vi "Print.vi"(5 "Orientation (0: Portrait)":i32(ring) items=["Portrait", "Landscape"], 7 "File Format (0: BMP)":i32(ring) items=["BMP", "Canon BubbleJet", "HP DeskJet", "Seiko DPU3445", "Seiko DPU411", "Seiko DPU412", "Epson C60", "Epson C80", "Epson Postscript", "Epson Dot Matrix", "Interleaf", "HP LaserJet II", "PCX", "RLE", "HP ThinkJet", "TIFF"], 8 "error in (no error)":errorcluster, 9 "Ink Saver (Off)":bool, 10 "Port (0: Centronics)":i32(ring) items=["Centronics", "Serial", "GPIB"], 11 "VISA resource name":refnum<visa-resource-name>) -> (0 "error out":errorcluster, 3 "VISA resource name out":refnum<visa-resource-name>)   [LabVIEW 2017, in "Tektronix TDS 200 1000 2000 Series.lvlib"]
doc: "Sets the format, orientation, and port for hardcopy printing."
uses:
  Tektronix TDS 200 1000 2000 Series.lvlib
panel:
  # "On"
  # "Off"
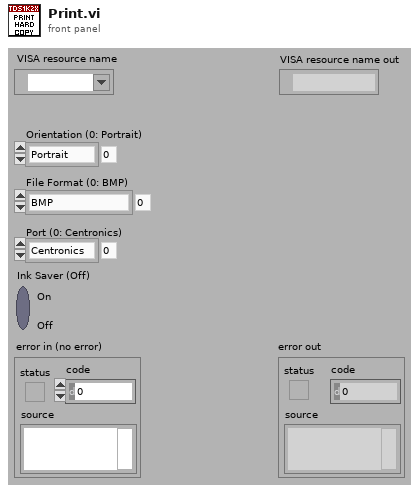
[diagram p1: front panel]
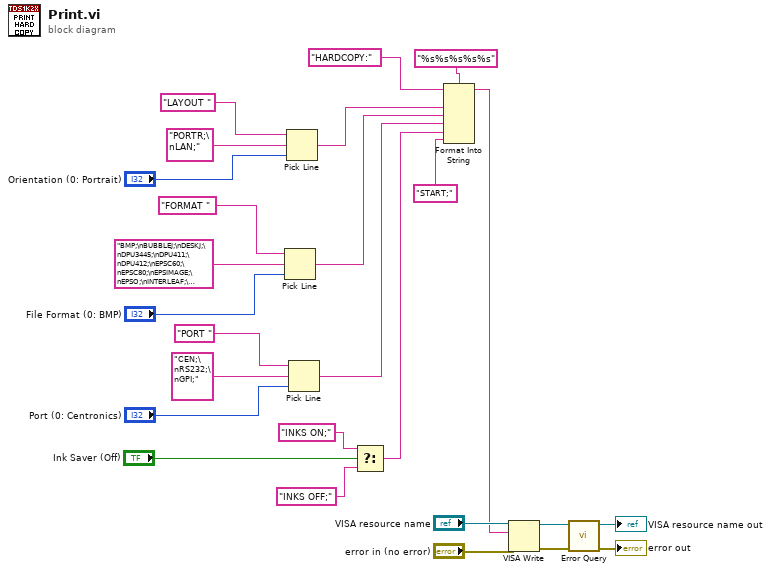
[diagram p0: block diagram]
diagram:
  n1 = Pick Line(string ("")="FORMAT ", multi-line string="BMP;\nBUBBLEJ;\nDESKJ;\nDPU3445;\nDPU411;\nDPU412;\nEPSC60;\nEPSC80;\nEPSIMAGE;\nEPSO;\nINTERLEAF;\nLASERJ;\nPCX;\nRLE;\nTHINK;\nTIFF;", line index="File Format (0: BMP)") -> (output string=w14:string)
  n2 = Pick Line(string ("")="LAYOUT ", multi-line string="PORTR;\nLAN;", line index="Orientation (0: Portrait)") -> (output string=w15:string)
  n3 = Pick Line(string ("")="PORT ", multi-line string="CEN;\nRS232;\nGPI;", line index="Port (0: Centronics)") -> (output string=w13:string)
  n4 = Select(t="INKS ON;", s="Ink Saver (Off)", f="INKS OFF;") -> (s? t:f=w9:string)
  n5 = Format Into String(format string="%s%s%s%s%s", initial string="HARDCOPY:", w15, w14, w13, w9, "START;") -> (resulting string=w2:string)  [unwired: 1 in, 1 out]
  n6 = VISA Write(VISA resource name="VISA resource name", write buffer=w2, error in (no error)="error in (no error)") -> (VISA resource name out=w7:refnum<visa-resource-name>, error out=w8:errorcluster)  [unwired: 1 out]
  n7 = call "Error Query.vi"("error in (no error)"=w8, "VISA resource name"=w7) -> ("error out"=→"error out":errorcluster, "VISA resource name out"=→"VISA resource name out":refnum<visa-resource-name>)  [unwired: 8 out]
